vi "2 Element Array FXP(+-,18,1) Remove Overflow.vi"(0 "data in":fxp<+/-,18,1>[](array[numeric])=[0.0, 0.0]) -> (4 "data out":fxp<+/-,18,1>[](array[numeric]), 6 "overflow":bool)   [LabVIEW 2014]
doc: "Removes and returns carried overflow from input data.\n\n<B>Supported data types</B>\nFXP +-,18,1; FXP +-,14,1\n\n<B>Supported channel size</B>\n4, 8\n\n<B>Supported samples per cycle</B>\n2\n\n<B>Input Parameters</B>\n\n<B>data in</B> specifies the data input carrying the overflow.\n\n<B>Output Parameters</B>\n\n<B>data out</B> returns the data without the overflow.\n\n<B>overflow</B> returns the overflow that was carried in the data input."
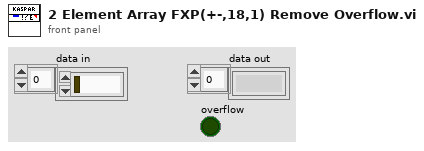
[diagram p1: front panel]
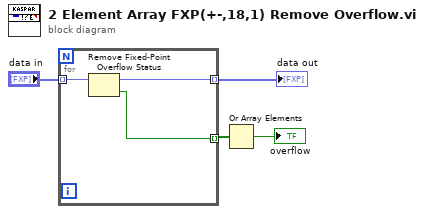
[diagram p0: block diagram]
diagram:
  n1 = for {
    tunnel: "data in" -> [w7] mode=indexing
    tunnel: [w5] -> w3 mode=indexing
    tunnel: [w6] -> w2 mode=indexing
    n2 = Remove Fixed-Point Overflow Status(3:w7) -> (0:w6:bool, 1:w5:fxp<+/-,18,1>)
  }
  "data out" <- w3
  n3 = Or Array Elements(Boolean array=w2) -> (logical OR=→"overflow":bool)
